vi "Main_11B.vi"() -> ()   [LabVIEW 2024]
uses:
  Map_Numbers to Counts.ctl
  <vilib>/Utility/miscctls.llb/LVMapReplaceAction.ctl
panel:
  out "Map":map{u64, u64}(c390)
  in  "Example 2":string="125 17"
  in  "Use Puzzle":bool
  out "Answer 228651922369703":u64
  in  "Puzzle":string="30 71441 3784 580926 2 8122942 0 291"
  in  "Example":string="0 1 10 99 999"
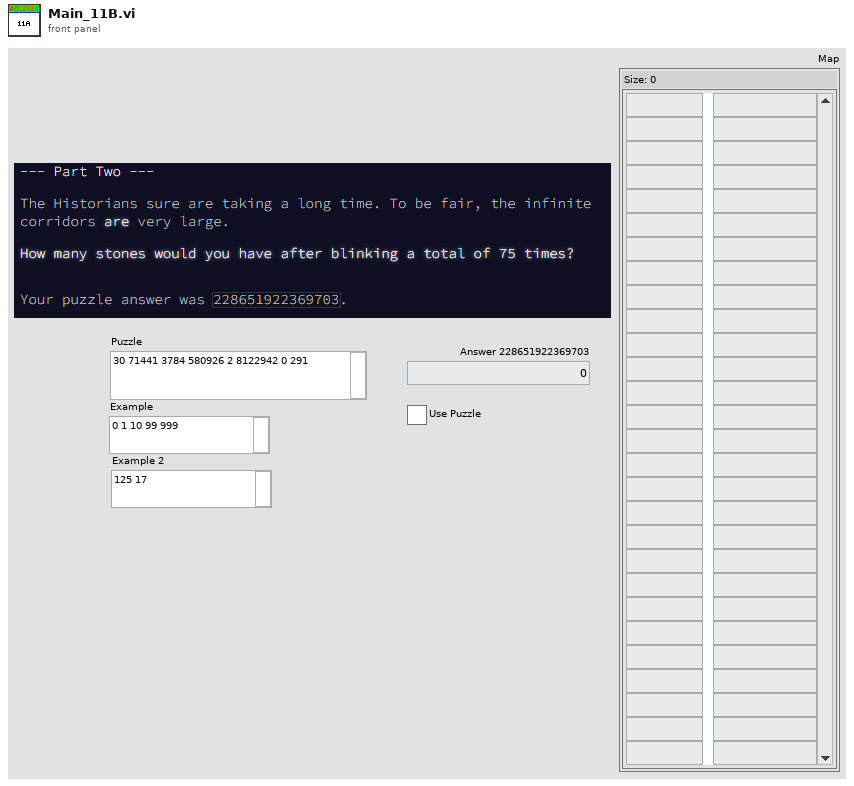
[diagram p1: front panel]
types:
  T1 = typedef "Map_Numbers to Counts.ctl" = map{u64, u64}
  T2 = typedef "LVMapReplaceAction.ctl" = enum32{"Modify Entry only if found", "Add or Modify Entry", "Delete Entry"}
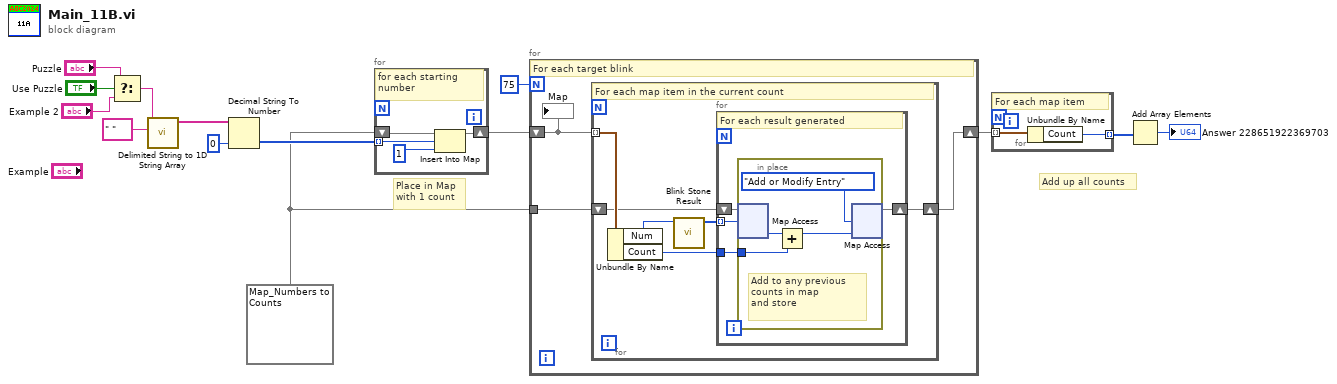
[diagram p0: block diagram]
diagram:
  w4 = T1 {}
  # "Add up all counts"
  # "Place in Map\nwith 1 count"
  n1 = Select(t="Puzzle", s="Use Puzzle", f="Example 2") -> (s? t:f=w12:string)
  n2 = call <vilib>:"Delimited String to 1D String Array.vi"("delimiter"=" " ("delimiter (Tab)"), "delimited string"=w12) -> ("string array"=w13:string[])  [unwired: 9 in]
  n3 = Decimal String To Number(string=w13, default (0L)=u64 0 ("default (0 I32)")) -> (number=w7:u64[])  [unwired: 1 in, 1 out]
  n4 = for {
    shift-right: [w17] -> w5
    shift-left: w4 -> [w18]
    tunnel: w7 -> [w16] mode=indexing
    # "for each starting number"
    n5 = Insert Into Map(map in=w18, key=w16, value=u64 1) -> (map out=w17:T1)  [unwired: 2 out]
  }
  n6 = for {
    N: 75 -> [_]
    shift-right: [w21] -> w3
    shift-left: w5 -> [w19]
    tunnel: w4 -> [w20]
    # "For each target blink"
    n7 = for {
      tunnel: w19 -> [w27] mode=indexing
      shift-right: [w23] -> w21
      shift-left: w20 -> [w25]
      # "For each map item in the current count"
      n8 = Unbundle By Name(w27) -> ("Num"=w22:u64, "Count"=w24:u64)
      n9 = call "Blink Stone Result.vi"("String"=w22) -> ("Result Array"=w26:u64[])  [unwired: 9 in, 1 out]
      n10 = for {
        tunnel: w26 -> [w29] mode=indexing
        shift-right: [w31] -> w23
        shift-left: w25 -> [w30]
        tunnel: w24 -> [w28]
        # "For each result generated"
        n11 = in-place {
          in-place-border: w28 -> [w33]
          # "Add to any previous\ncounts in map\nand store"
          n12 = in-place-map #1(w30, w29) -> (w34:u64)  [unwired: 1 in, 1 out]
          n13 = Add(x=w34, y=w33) -> (x+y=w32:u64)
          n14 = in-place-map #1(w32, LVMapReplaceAction."Add or Modify Entry" ("action")) -> (w31:T1)  [unwired: 2 out]
        }
      }
    }
    "Map" <- w19
  }
  n15 = for {
    tunnel: w3 -> [w37] mode=indexing
    tunnel: [w36] -> w2 mode=indexing
    # "For each map item"
    n16 = Unbundle By Name(w37) -> ("Count"=w36:u64)
  }
  n17 = Add Array Elements(numeric array=w2) -> (sum=→"Answer 228651922369703":u64)
